vi "Prepare Statement.vi"(8 "error in (no error)":errorcluster, 10 "Statement in":string="INSERT INTO myTable VALUES(NULL, @number, @text)", 11 "mysql in":refnum<class "mysql.lvclass">) -> (0 "error out":errorcluster, 2 "Numeric":u64, 3 "mysql out":refnum<class "mysql.lvclass">)   [LabVIEW 2020, in "mysql.lvlib" / "mysql.lvclass"]
uses:
  mysql.lvclass
  MySql.Data
  mysql.lvclass/mysql.ctl
panel:
  out "MySqlCommand out":refnum<k24>
  # "Implementation may change this connector pane.\nThis is just a guess."
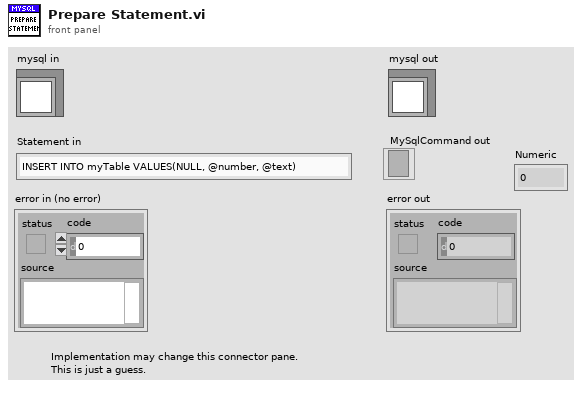
[diagram p1: front panel]
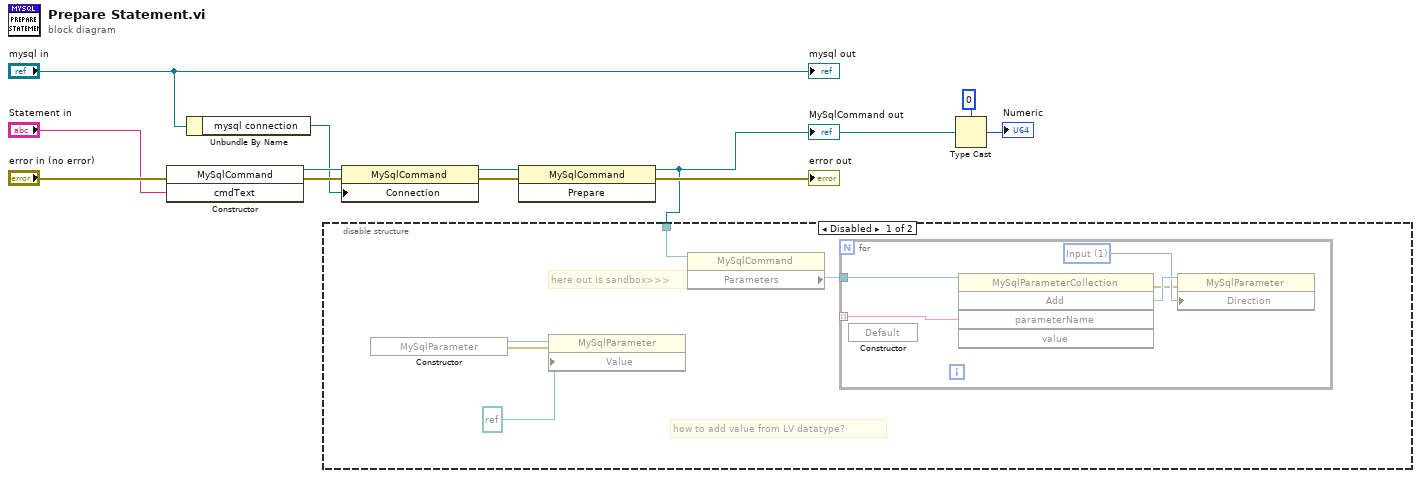
[diagram p0: block diagram]
diagram:
  n1 = constructor class="MySqlCommand"(error in="error in (no error)", "cmdText"="Statement in") -> (reference out=w9:refnum<k24>, error out=w10:errorcluster)  [unwired: 2 in, 2 out]
  n2 = Unbundle By Name("mysql in") -> ("mysql connection"=w8:refnum<k24>)
  n3 = property class="MySqlCommand"(reference=w9, error in=w10, "Connection"=w8) -> (reference out=w6:refnum<k24>, error out=w7:errorcluster)
  n4 = invoke class="MySqlCommand" method="Prepare"(reference=w6, error in=w7) -> (reference out=w4:refnum<k24>, error out=→"error out":errorcluster)  [unwired: 1 in, 1 out]
  "MySqlCommand out" <- w4
  n5 = disable-structure shown="Disabled" {
    disable-tunnel: w4 -> [w18 _]
    frame Disabled {
      # "how to add value from LV datatype?"
      # "here out is sandbox>>>"
      n6 = constructor class="MySqlParameter"() -> (reference out=w15:refnum<k24>, error out=w14:errorcluster)  [unwired: 3 in, 1 out]
      n7 = property class="MySqlParameter"(reference=w15, error in=w14, "Value"=refnum<k24> refnum) -> ()  [unwired: 2 out]
      n8 = property class="MySqlCommand"(reference=w18) -> ("Parameters"=w17:refnum<k24>)  [unwired: 1 in, 2 out]
      n9 = for {
        tunnel: w17 -> [w23]
        tunnel: [w19] -> w16 mode=indexing
        w21 = 1 items=["Input"=1, "Output"=2, "InputOutput"=3, "ReturnValue"=6] ("Direction")
        n10 = constructor class=".NET"() -> ()  [unwired: 3 in, 3 out]
        n11 = invoke class="MySqlParameterCollection" method="Add"(reference=w23, "parameterName"=w19) -> (error out=w20:errorcluster, "Add"=w22:refnum<k24>)  [unwired: 3 in, 3 out]
        n12 = property class="MySqlParameter"(reference=w22, error in=w20, "Direction"=w21) -> ()  [unwired: 2 out]
      }
    }
    frame Enabled {
    }
  }
  n13 = Type Cast(type=u64 0 ("Numeric 2"), x=w4) -> (*(type *) &x=→"Numeric":u64)
  "mysql out" <- "mysql in"
